vi "Configure Channel Input.vi"(5 "Enable Filter (Disable)":bool, 6 "Impedance (1E+6 OHM)":i32(ring)=1000000 items=["1E+6"=1000000, "50"=50], 7 "Channel (1:Channel 1)":i32(ring)=1 items=["Channel 1"=1, "Channel 2"=2], 8 "error in (no error)":errorcluster, 9 "Attenuation (1)":u16(ring)=1 items=["1"=1, "10"=10], 10 "Coupling (0:AC)":i32(ring) items=["AC", "DC"], 11 "VISA resource name":refnum<visa-resource-name>) -> (0 "error out":errorcluster, 3 "VISA resource name out":refnum<visa-resource-name>)   [LabVIEW 2020, in "Counter.lvlib" / "PICOTEST U62XXA series.lvlib"]
doc: "Configures the characteristics of the channel to which an input is connected."
uses:
  PICOTEST U62XXA series.lvlib
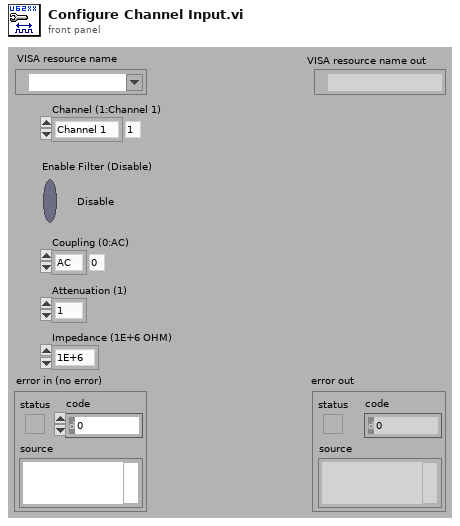
[diagram p1: front panel]
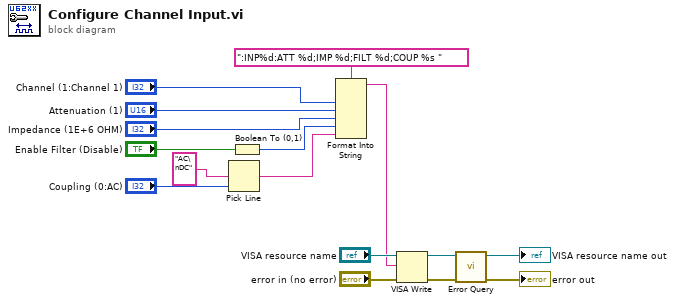
[diagram p0: block diagram]
diagram:
  n1 = Pick Line(multi-line string="AC\nDC" ("format string"), line index="Coupling (0:AC)") -> (output string=w4:string)  [unwired: 1 in]
  n2 = Boolean To (0,1)(Boolean="Enable Filter (Disable)") -> (0, 1=w11:i16)
  n3 = Format Into String(format string=":INP%d:ATT %d;IMP %d;FILT %d;COUP %s ", "Channel (1:Channel 1)", "Attenuation (1)", "Impedance (1E+6 OHM)", w11, w4) -> (resulting string=w12:string)  [unwired: 2 in, 1 out]
  n4 = VISA Write(VISA resource name="VISA resource name", write buffer=w12, error in (no error)="error in (no error)") -> (VISA resource name out=w10:refnum<visa-resource-name>, error out=w8:errorcluster)  [unwired: 1 out]
  n5 = call "Error Query.vi"("error in (no error)"=w8, "VISA resource name"=w10) -> ("error out"=→"error out":errorcluster, "VISA resource name out"=→"VISA resource name out":refnum<visa-resource-name>)  [unwired: 6 in, 2 out]
